vi "AutoChargeTiming.vi"(2 "Auto Charge In":bool caption="Charge\nForm", 3 "Timeout (s)":dbl=180.0, 4 "Shot Period (s)":dbl=180.0, 5 "Time Since Last Shot":dbl=334895.7833442688 step=8.0 format="%<%H:%M:%S>t") -> (0 "Auto Charge Out":bool caption="Charge\nForm", 1 "Time to charge":bool)   [LabVIEW 2009]
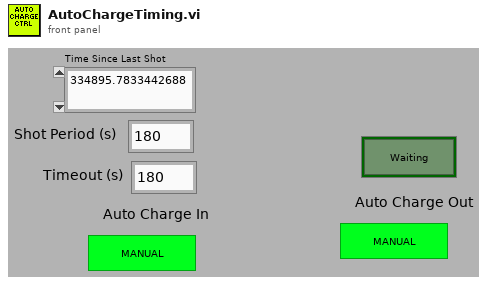
[diagram p1: front panel]
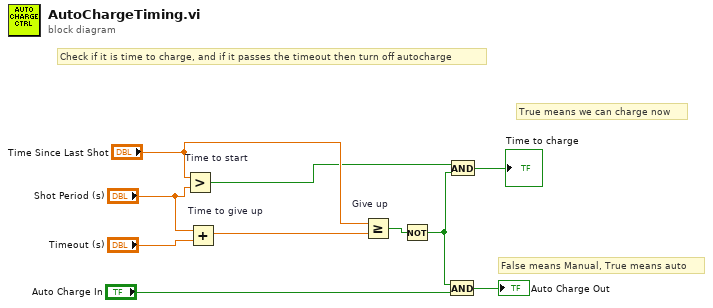
[diagram p0: block diagram]
diagram:
  # "Check if it is time to charge, and if it passes the timeout then turn off autocharge"
  # "True means we can charge now"
  # "False means Manual, True means auto"
  n1 = Greater? "Time to start"(x="Time Since Last Shot", y="Shot Period (s)") -> (0:w1:bool)
  n2 = Add "Time to give up"(x="Shot Period (s)", y="Timeout (s)") -> (x+y=w8:dbl)
  n3 = Greater Or Equal? "Give up"(x="Time Since Last Shot", y=w8) -> (x >= y?=w5:bool)
  n4 = Not(x=w5) -> (.not. x?=w3:bool)
  n5 = And(x=w3, y="Auto Charge In") -> (x .and. y?=→"Auto Charge Out":bool)
  n6 = And(x=w1, y=w3) -> (x .and. y?=→"Time to charge":bool)
